vi "KB-CalOffsetAndFlatness - 副本.vi"(0 "Image In":T1(plugin-control), 1 "Src Data":dbl[][](array[numeric]), 5 "ROI Descriptor":T2 {"Contours"."Type" items=["No Selection", "Point", "Line", "Rectangle", "Oval", "Polygon", "Freehand Region", "Annulus", "Unused2", "Unused3", "Broken Line", "Freehand Line", "Rotated Rectangle"]}, 9 "y":dbl=200.0 format="%#_13g", 11 "error in (no error)":errorcluster) -> (3 "New Cent":dbl[](array[numeric]), 4 "Image Out":T1(plugin-control), 8 "子数组":dbl[][](array[numeric]), 10 "Point":cluster{"X":dbl, "Y":dbl, "Z":dbl}[](array[cluster]), 15 "error Out (no error)":errorcluster)   [LabVIEW 2015]
uses:
  <vilib>/Math Plots/3D Math Plots/3D Surface/3D Surface XCtrl/3D Surface.xctl
  <vilib>/Math Plots/3D Math Plots/3D Surface/3D Surface Datatype/Public/Plot Helper (Matrix).vi
  <vilib>/Math Plots/3D Math Plots/3D Surface/3D Surface Datatype/3D Surface Datatype.lvclass
panel:
  out "MIX Y":dbl
  out "MIX X":dbl
  out "MAX X":dbl
  out "MAX Y":dbl
  out "最小值":dbl
  out "最大值 2":dbl
  out "3D Surface 2":refnum<class "3D Plot Datatype.lvclass">[](xcontrol) caption="三维曲面"
  out "Point min":cluster{"X":dbl, "Y":dbl, "Z":dbl}[](array[cluster])
  out "数值 5":i32
  out "数值 4":i32
  out "3D Surface Old 2":refnum<class "3D Plot Datatype.lvclass">[](xcontrol) caption="三维曲面"
  out "Coordinates 2":i32[](array[numeric])
  out "3D Surface":refnum<class "3D Plot Datatype.lvclass">[](xcontrol) caption="三维曲面"
  out "Radius (Pixels)":dbl
  out "Image Out 3":T1(plugin-control)
  out "Image Out 2":T1(plugin-control)
  out "数组":dbl[](array[numeric])
  out "行数":dbl
  out "列数":dbl
  out "最大值":dbl
  out "Y Resolution":i32
  out "X Resolution":i32
  out "Y":i32
  out "X":i32
  out "Coordinates":i32[](array[numeric])
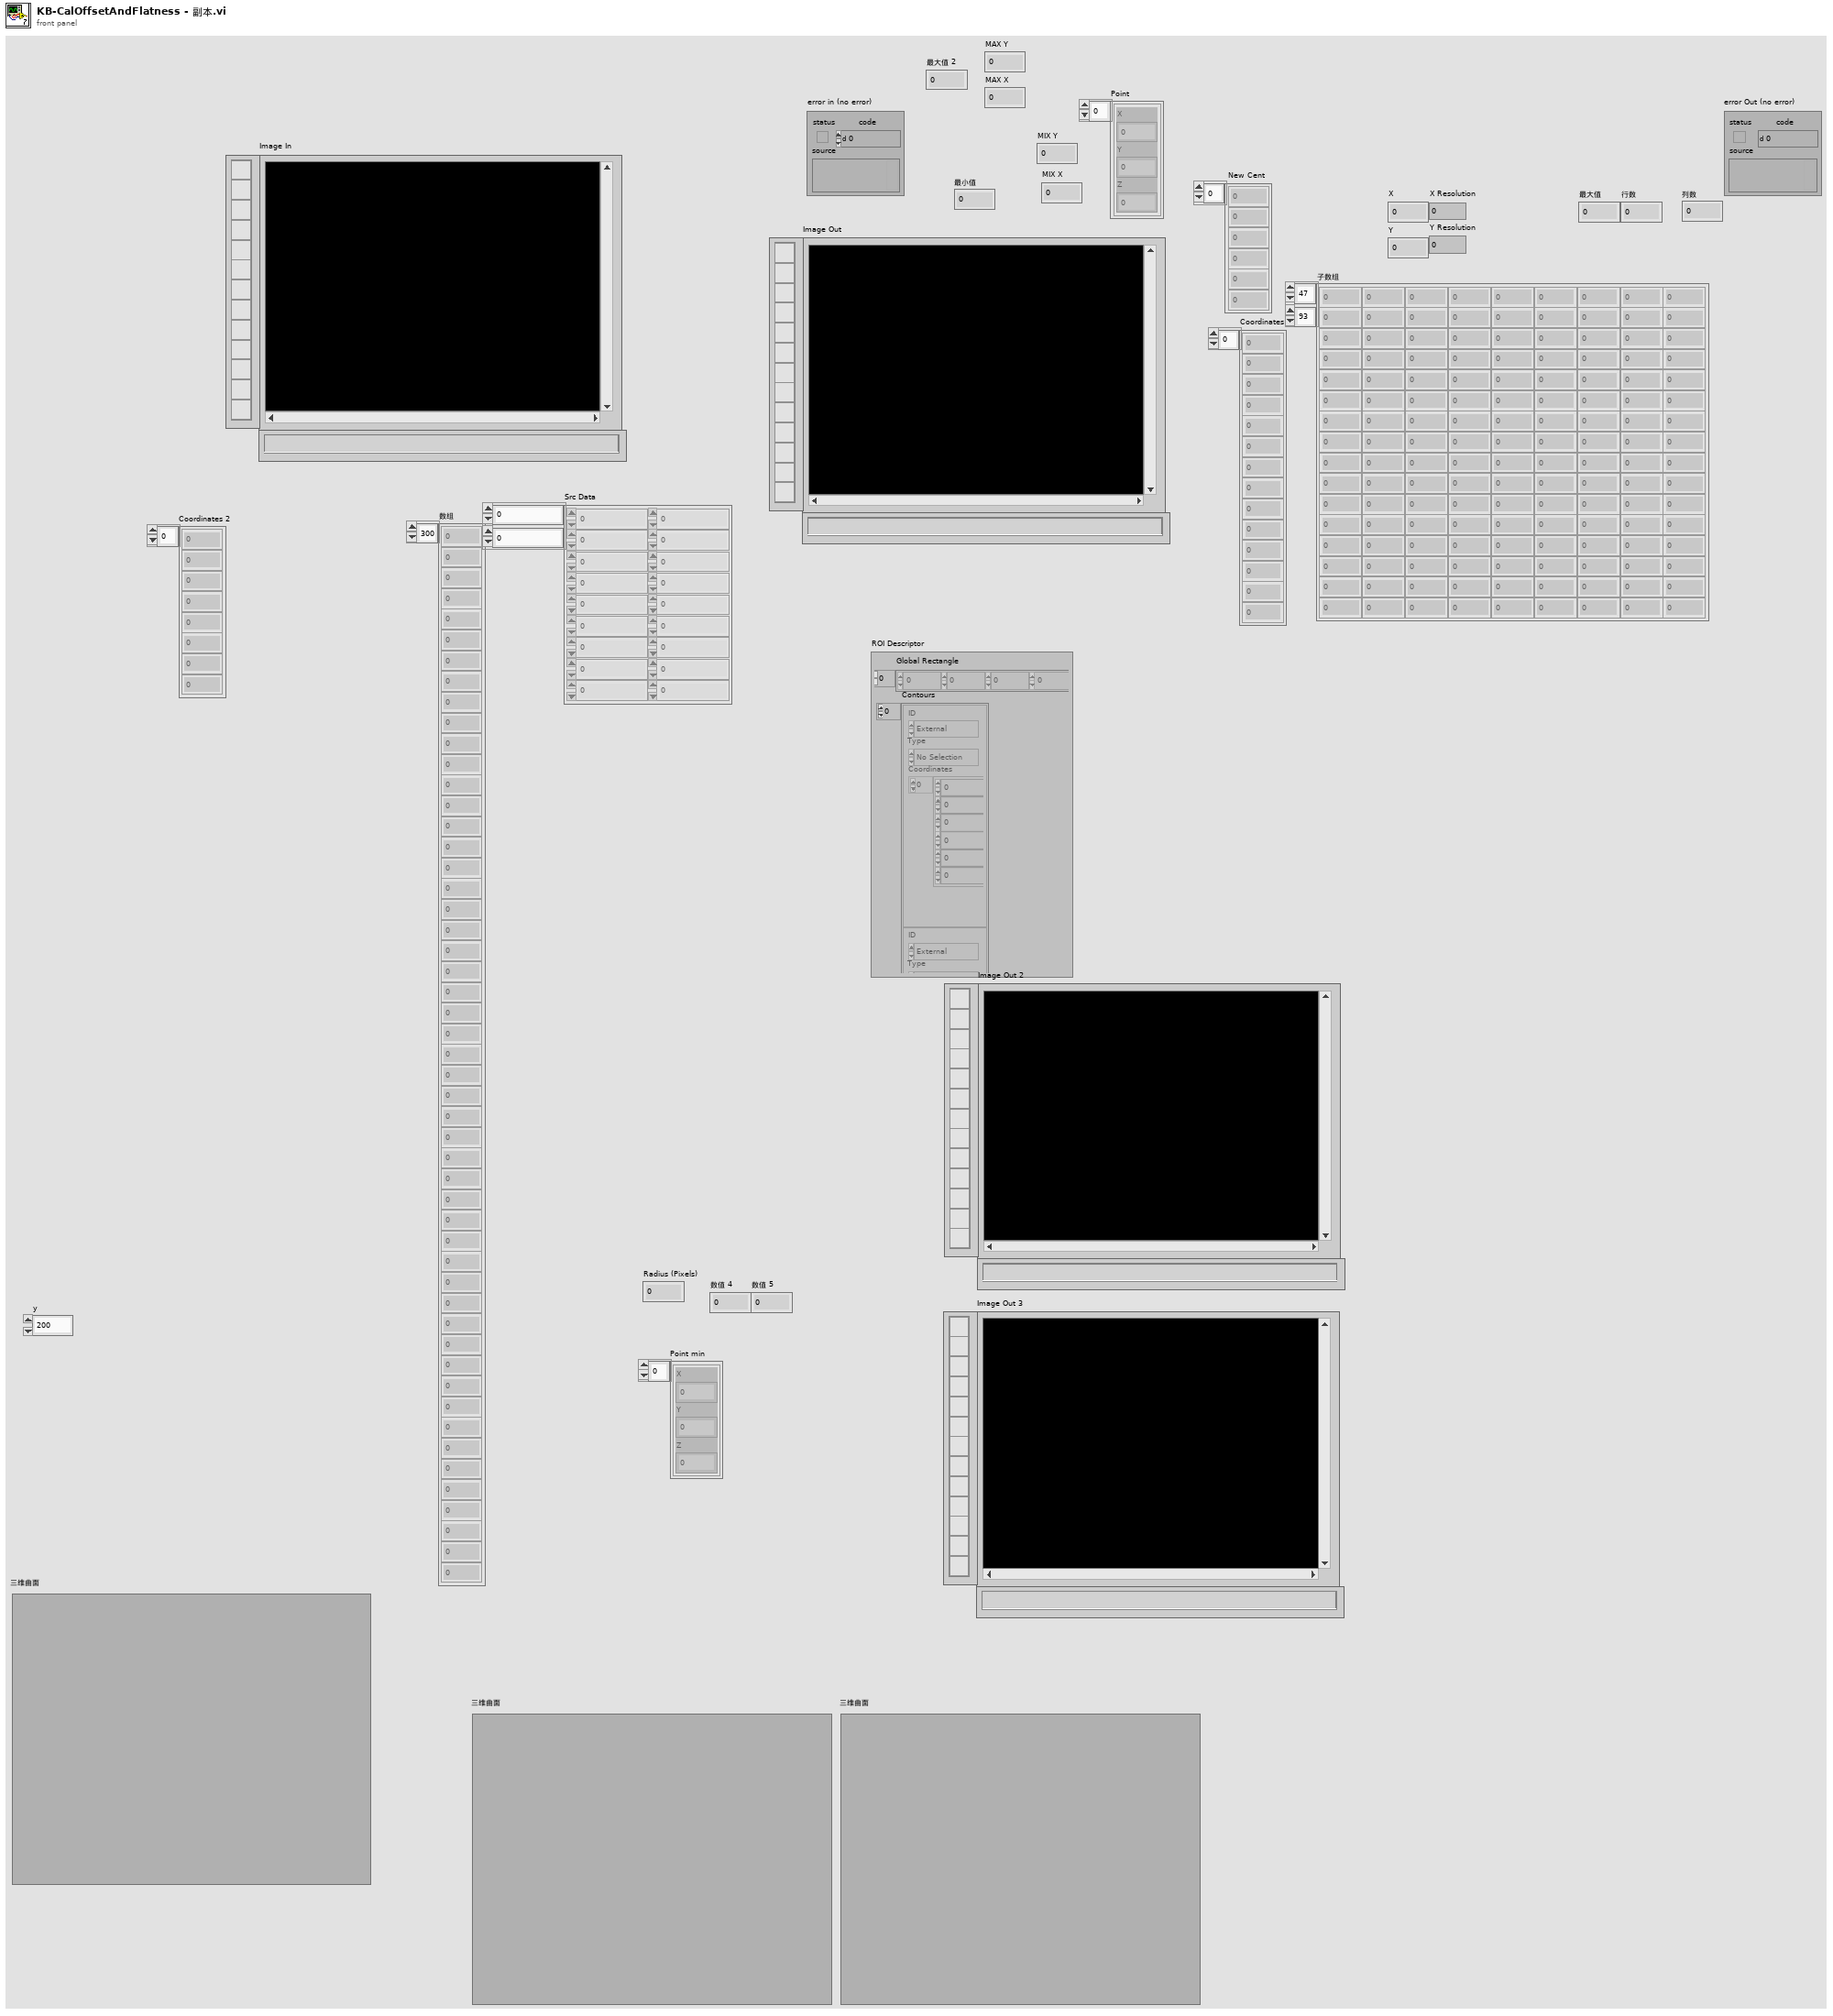
[diagram p1: front panel]
types:
  T1 = typedef "IMAQ Image.ctl" = refnum<image>
  T2 = typedef "ROI Descriptor" = cluster{"Global Rectangle":i32[], "Contours":cluster{"ID":enum32{"External", "Internal"}, "Type":u32, "Coordinates":i32[]}[]}
  T3 = typedef "IMAQ Circle" = cluster{"Center X":i32, "Center Y":i32, "Inner Radius":i32, "Outer Radius":i32, "Start Angle":dbl, "End Angle":dbl}
  T4 = cluster{"ID":enum32{"External", "Internal"}, "Type":u32, "Coordinates":i32[]}[]
  T5 = cluster{"ID":enum32{"External", "Internal"}, "Type":u32, "Coordinates":i32[]}
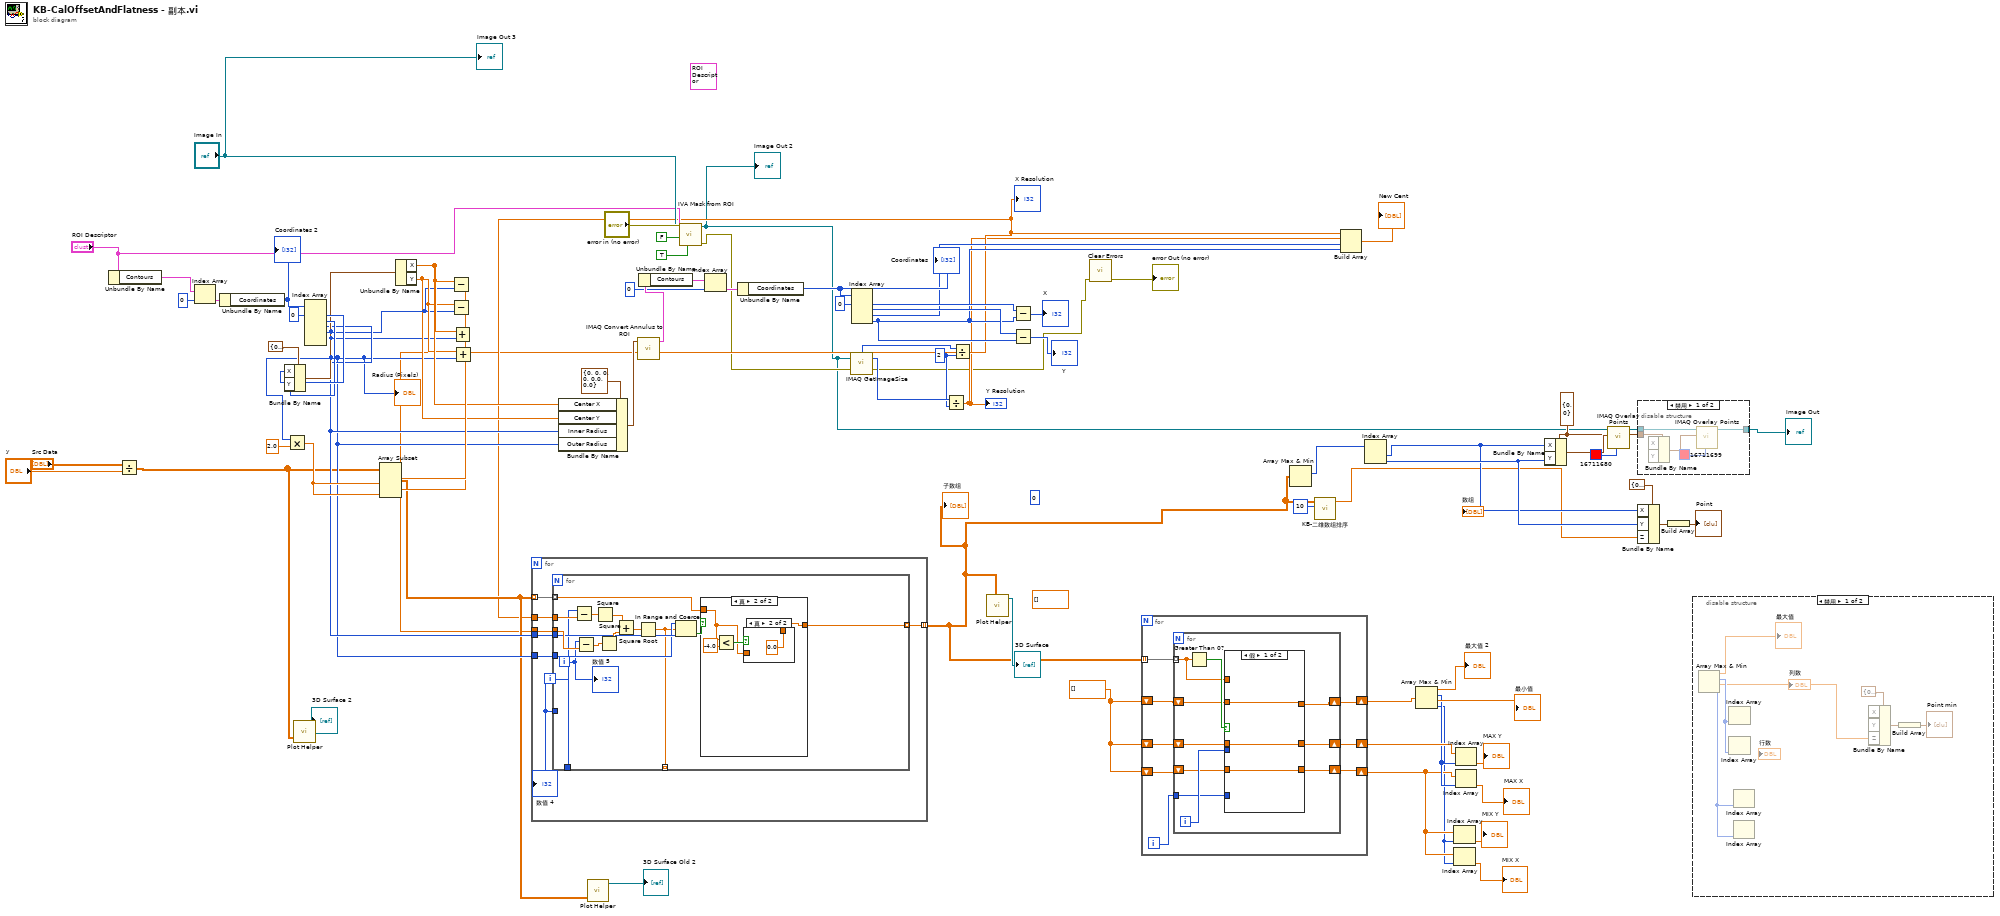
[diagram p0: block diagram]
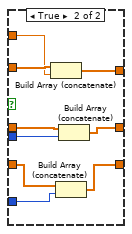
[diagram p2: hidden frame]
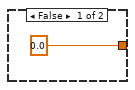
[diagram p5: hidden frame]
diagram:
  w17 = dbl[] []
  w22 = cluster{"X":i32, "Y":i32} {"X"=0, "Y"=0} ("Point")
  (unwired) 0
  (unwired) dbl[] []
  w73 = 2 ("y")
  (unwired) T2 {"Global Rectangle"=[-1, -1, 2, 2], "Contours"=[{"ID"=enum."External", "Type"=7, "Coordinates"=[0, 0, 0, 0, 0, 0]}]} ("ROI Descriptor")
  n1 = Unbundle By Name("ROI Descriptor") -> ("Contours"=w49:T4)
  n2 = Divide(x="Src Data", y="y") -> (x/y=w20:dbl[][])
  n3 = Index Array(array=w49, index=0 ("索引")) -> (element=w46:T5)
  n4 = Unbundle By Name(w46) -> ("Coordinates"=w45:i32[])
  "Coordinates 2" <- w45
  n5 = call-poly <vilib>:"Plot Helper.vi"("z matrix"=w20) -> ("3D Plot lvclass Array out"=→"3D Surface 2":refnum<class "3D Plot Datatype.lvclass">[])  [unwired: 5 in, 5 out]
  n6 = Index Array(array=w45, index #1=0 ("索引")) -> (element #1=w42:i32, element #2=w41:i32, element #3=w34:i32, element #4=w33:i32)  [unwired: 5 in, 2 out]
  "Radius (Pixels)" <- w33
  n7 = Bundle By Name(cluster=cluster{"Y":dbl, "X":dbl} {"Y"=0.0, "X"=0.0}, "X"=w42, "Y"=w41) -> (w40:cluster{"Y":dbl, "X":dbl})
  n8 = Multiply(x=w33, y=2.0) -> (x*y=w51:dbl)
  n9 = Unbundle By Name(w40) -> ("X"=w36:dbl, "Y"=w35:dbl)
  n10 = Subtract(x=w36, y=w33) -> (x-y=w38:dbl)
  n11 = Subtract(x=w35, y=w33) -> (x-y=w50:dbl)
  n12 = Array Subset(array=w20, index (row)=w50, length (row)=w51, index (col)=w38, length (col)=w51) -> (w32:dbl[][])
  n13 = Add(x=w36, y=w33) -> ()  [unwired: 1 out]
  n14 = Add(x=w35, y=w33) -> ()  [unwired: 1 out]
  n15 = Bundle By Name(cluster=T3 {"Center X"=0, "Center Y"=0, "Inner Radius"=0, "Outer Radius"=0, "Start Angle"=0.0, "End Angle"=0.0} ("Annulus"), "Center X"=w36, "Center Y"=w35, "Inner Radius"=w34, "Outer Radius"=w33) -> (w60:T3)
  n16 = call-poly <vilib>:"Plot Helper.vi"("z matrix"=w32) -> ("3D Plot lvclass Array out"=→"3D Surface Old 2":refnum<class "3D Plot Datatype.lvclass">[])  [unwired: 5 in, 5 out]
  n17 = call "IMAQ Convert Annulus to ROI"("Annulus"=w60) -> ("ROI Descriptor"=w59:T2)  [unwired: 8 in, 1 out]
  n18 = Unbundle By Name(w59) -> ("Contours"=w56:T4)
  n19 = call <vilib>:"IVA Mask from ROI.vi"("Shrink"=TRUE, "ROI Descriptor"="ROI Descriptor", "error in (no error)"="error in (no error)", "Out / In"=FALSE, "Image Src"="Image In") -> ("error out"=w28:errorcluster, "Image Out"=w18:T1)  [unwired: 5 out]
  "Image Out 2" <- w18
  n20 = Index Array(array=w56, index=0 ("索引")) -> (element=w54:T5)
  n21 = Unbundle By Name(w54) -> ("Coordinates"=w79:i32[])
  "Coordinates" <- w79
  n22 = call "IMAQ GetImageSize"("Image"=w18, "error in (no error)"=w28) -> ("Y Resolution"=w74:i32, "X Resolution"=w75:i32, "error out"=w27:errorcluster)  [unwired: 2 in]
  n23 = Index Array(array=w79, index #1=0 ("索引")) -> (element #1=w77:i32, element #2=w76:i32, element #3=w69:i32, element #4=w68:i32)  [unwired: 3 in]
  n24 = Divide(x=w74, y=w73) -> (x/y=w30:dbl)
  "Y Resolution" <- w30
  n25 = Divide(x=w75, y=w73) -> (x/y=w31:dbl)
  "X Resolution" <- w31
  n26 = for {
    tunnel: w32 -> [w82] mode=indexing
    tunnel: w31 -> [w86]
    tunnel: w30 -> [w85]
    tunnel: w34 -> [w84]
    tunnel: w33 -> [w83]
    tunnel: [w81] -> w3 mode=indexing
    i -> [w80]
    n27 = for {
      tunnel: w86 -> [w101]
      tunnel: w85 -> [w100]
      tunnel: w80 -> [w87]
      tunnel: w84 -> [w94]
      tunnel: w83 -> [w93]
      tunnel: w82 -> [w91] mode=indexing
      tunnel: [w88] -> w81 mode=indexing
      tunnel: [w89] -> _ mode=indexing
      tunnel: w80 -> [_]
      i -> [w90]
      n28 = Subtract(x=w87, y=w101) -> (x-y=w99:dbl)
      n29 = Subtract(x=w90, y=w100) -> (x-y=w98:dbl)
      n30 = Square(x=w99) -> (x^2=w97:dbl)
      n31 = Square(x=w98) -> (x^2=w96:dbl)
      n32 = Add(x=w97, y=w96) -> (x+y=w95:dbl)
      n33 = Square Root(x=w95) -> (sqrt(x)=w89:dbl)
      n34 = In Range and Coerce(upper limit=w93, x=w89, lower limit=w94) -> (In Range?=w92:bool)  [unwired: 1 out]
      n35 = case shown="真" w92 {
        tunnel: w91 -> [_ w104]
        tunnel: [0.0 w103] -> w88
        frame False {
        }
        frame True {
          n36 = Less?(x=w104, y=-4.0) -> (x < y?=w105:bool)
          n37 = case shown="真" w105 {
            tunnel: w104 -> [w107 _]
            tunnel: [w107 0.0 ("y")] -> w103
            frame False {
            }
            frame True {
            }
          }
        }
      }
      "数值 5" <- w90
    }
    "数值 4" <- w80
  }
  "子数组" <- w3
  n38 = call-poly <vilib>:"Plot Helper.vi"("z matrix"=w3) -> ("3D Plot lvclass Array out"=→"3D Surface":refnum<class "3D Plot Datatype.lvclass">[])  [unwired: 5 in, 5 out]
  n39 = Subtract(x=w77, y=w68) -> (x-y=→"X":i32)
  n40 = Subtract(x=w76, y=w68) -> (x-y=→"Y":i32)
  n41 = call <vilib>:"Clear Errors.vi"("error in (no error)"=w27) -> ("error out"=→"error Out (no error)":errorcluster)  [unwired: 5 in, 1 out]
  n42 = for {
    tunnel: w3 -> [w116] mode=indexing
    shift-right: [w114] -> w16
    shift-left: w17 -> [w115]
    shift-right: [w112] -> w13
    shift-left: w17 -> [w113]
    shift-right: [w110] -> w7
    shift-left: w17 -> [w111]
    i -> [w109]
    n43 = for {
      tunnel: w116 -> [w124] mode=indexing
      shift-right: [w123] -> w114
      shift-left: w115 -> [w125]
      shift-right: [w120] -> w112
      shift-left: w113 -> [w121]
      shift-right: [w117] -> w110
      shift-left: w111 -> [w119]
      tunnel: w109 -> [w118]
      i -> [w122]
      n44 = Greater Than 0?(x=w124) -> (x > 0?=w126:bool)
      n45 = case shown="假" w126 {
        tunnel: w125 -> [w129 w138]
        tunnel: w124 -> [_ w137]
        tunnel: [w129 w136] -> w123
        tunnel: w122 -> [_ w135]
        tunnel: w121 -> [w128 w134]
        tunnel: [w128 w133] -> w120
        tunnel: w119 -> [w127 w131]
        tunnel: w118 -> [_ w132]
        tunnel: [w127 w130] -> w117
        frame False {
        }
        frame True {
          n46 = Build Array (concatenate)(w138, w137) -> (w136:dbl[])
          n47 = Build Array (concatenate)(w131, w132) -> (w130:dbl[])
          n48 = Build Array (concatenate)(w134, w135) -> (w133:dbl[])
        }
      }
    }
  }
  n49 = Array Max & Min(array=w3) -> (max index (indices)=w19:i32[])  [unwired: 3 out]
  n50 = call "KB-二维数组排序.vi"("平均个数"=10, "二维数组"=w3) -> ("平均最高值"=w1:dbl)  [unwired: 9 in]
  n51 = Build Array(w31, w30, w69, w68) -> (→"New Cent":dbl[])
  n52 = Index Array(array=w19) -> (element #1=w4:i32, element #2=w5:i32)  [unwired: 2 in]
  n53 = Array Max & Min(array=w16) -> (max value=→"最大值 2":dbl, max index (indices)=w12:i32, min value=→"最小值":dbl, min index (indices)=w6:i32)
  n54 = Index Array(array=w7, index=w6) -> (element=→"MIX Y":dbl)
  n55 = Index Array(array=w7, index=w6) -> (element=→"MIX X":dbl)
  n56 = Index Array(array=w13, index=w12) -> (element=→"MAX Y":dbl)
  n57 = Index Array(array=w7, index=w12) -> (element=→"MAX X":dbl)
  n58 = Bundle By Name(cluster=w22, "X"=w4, "Y"=w5) -> (w71:cluster{"X":i32, "Y":i32})
  n59 = call "IMAQ Overlay Points"("Color"=u32 16711680, "Point"=w71, "Image"=w18) -> ("Image Out"=w24:T1)  [unwired: 7 in, 1 out]
  n60 = disable-structure shown="禁用" {
    disable-tunnel: w24 -> [w142 w144]
    disable-tunnel: [w141 w144] -> w23
    disable-tunnel: w22 -> [w140 _]
    frame Disabled {
      n61 = Bundle By Name(cluster=w140) -> (w139:cluster{"X":i32, "Y":i32})  [unwired: 2 in]
      n62 = call "IMAQ Overlay Points"("Color"=u32 16711699, "Point"=w139, "Image"=w142) -> ("Image Out"=w141:T1)  [unwired: 7 in, 1 out]
    }
    frame Enabled {
    }
  }
  "Image Out" <- w23
  n63 = Bundle By Name(cluster=cluster{"X":dbl, "Y":dbl, "Z":dbl} {"X"=0.0, "Y"=0.0, "Z"=0.0}, "X"=w4, "Y"=w5, "Z"=w1) -> (w65:cluster{"X":dbl, "Y":dbl, "Z":dbl})
  n64 = Build Array(w65) -> (→"Point":cluster{"X":dbl, "Y":dbl, "Z":dbl}[])
  n65 = disable-structure shown="禁用" {
    frame Disabled {
      n66 = Array Max & Min() -> (max value=→"最大值":dbl, max index (indices)=w151:i32, min value=w146:dbl, min index (indices)=w145:i32)  [unwired: 1 in]
      n67 = Index Array(index=w151) -> ()  [unwired: 1 in, 1 out]
      n68 = Index Array(index=w151) -> ()  [unwired: 1 in, 1 out]
      n69 = Index Array(index=w145) -> ()  [unwired: 1 in, 1 out]
      n70 = Index Array(index=w145) -> ()  [unwired: 1 in, 1 out]
      n71 = Bundle By Name(cluster=cluster{"X":dbl, "Y":dbl, "Z":dbl} {"X"=0.0, "Y"=0.0, "Z"=0.0}, "Z"=w146) -> (w148:cluster{"X":dbl, "Y":dbl, "Z":dbl})  [unwired: 2 in]
      n72 = Build Array(w148) -> (→"Point min":cluster{"X":dbl, "Y":dbl, "Z":dbl}[])
    }
    frame Enabled {
    }
  }
  "Image Out 3" <- "Image In"
